vi "Wait for Framework Command.vi"(8 "error in (no error)":errorcluster, 9 "timeout in ms (5000)":i32=5000 format="%d ms", 11 "Dispatcher in":refnum<class "Dispatcher Thread.lvclass">) -> (0 "error out":errorcluster, 2 "command":T1={"Command"=enum."Rx", "Parameters"={"arg1"=0, "arg2"=0}}, 3 "Dispatcher out":refnum<class "Dispatcher Thread.lvclass">)   [LabVIEW 2017, in "DSF Core.lvlib" / "Dispatcher Thread.lvclass"]
uses:
  Dispatcher Thread.lvclass
  Interface/Dispatcher/Command Data.ctl
  Interface/Dispatcher/Command.ctl
  Interface/Dispatcher/Parameters.ctl
  Dispatcher Thread.lvclass/Dispatcher Thread.ctl
  Interface/Dispatcher/Dispatcher Interface.lvclass
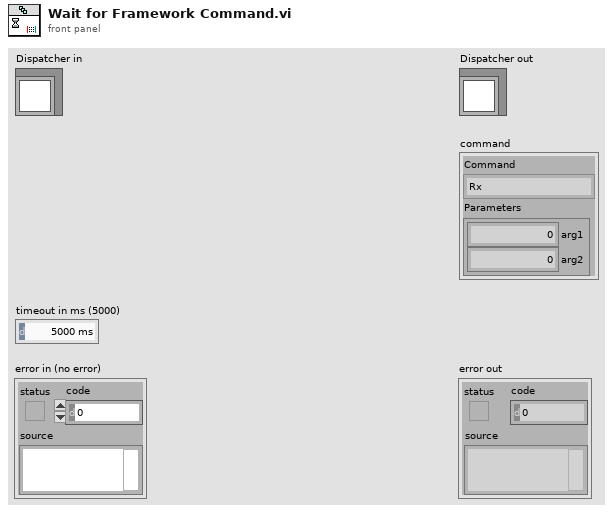
[diagram p1: front panel]
types:
  T1 = typedef "DSF Core.lvlib/Dispatcher Interface.lvclass/Command Data.ctl" = cluster{"Command":T2, "Parameters":T3}
  T2 = typedef "DSF Core.lvlib/Dispatcher Interface.lvclass/Command.ctl" = enum8{"Idle", "Start", "Rx", "Tx", "Set Inline Buffer", "Shutdown", "Error"}
  T3 = typedef "DSF Core.lvlib/Dispatcher Interface.lvclass/Parameters.ctl" = cluster{"arg1":u64, "arg2":u64}
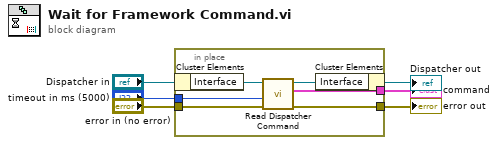
[diagram p0: block diagram]
diagram:
  n1 = in-place {
    in-place-border: "timeout in ms (5000)" -> [w12]
    in-place-border: "error in (no error)" -> [w11]
    in-place-border: [w10] -> w2
    in-place-border: [w9] -> w1
    n2 = in-place-cluster #1("Dispatcher in") -> ("Interface"=w8:refnum<class "Dispatcher Interface.lvclass">)
    n3 = call "Read Dispatcher Command.vi"("error in (no error)"=w11, "timeout in ms (0)"=w12, "Dispatcher Interface in"=w8) -> ("error out"=w10:errorcluster, "command"=w9:T1, "Dispatcher Interface out"=w7:refnum<class "Dispatcher Interface.lvclass">)  [unwired: 5 in, 1 out]
    n4 = in-place-cluster #1("Interface"=w7) -> (→"Dispatcher out":refnum<class "Dispatcher Thread.lvclass">)
  }
  "error out" <- w2
  "command" <- w1
